vi "Insert Path Node.vi"(7 "MulticolumnListbox in":refnum<vi>, 8 "ID":i16, 9 "Node To Index Lookup Map in":map{i16, i16[]}(c390), 10 "Tree":T2[](array[typedef]), 11 "CellPosition":T1) -> (1 "Index of Selected Node":i32, 2 "Tree Out":T2[](array[typedef]), 3 "Node To Index Lookup Map out":map{i16, i16[]}(c390))   [LabVIEW 2025]
uses:
  Types/Sequencing Tree Node.ctl
  Types/Single Cmd Info.ctl
  <vilib>/picture/picture.llb/imagedata.ctl
  <vilib>/Utility/miscctls.llb/LVRowAndColumnTypeDef.ctl
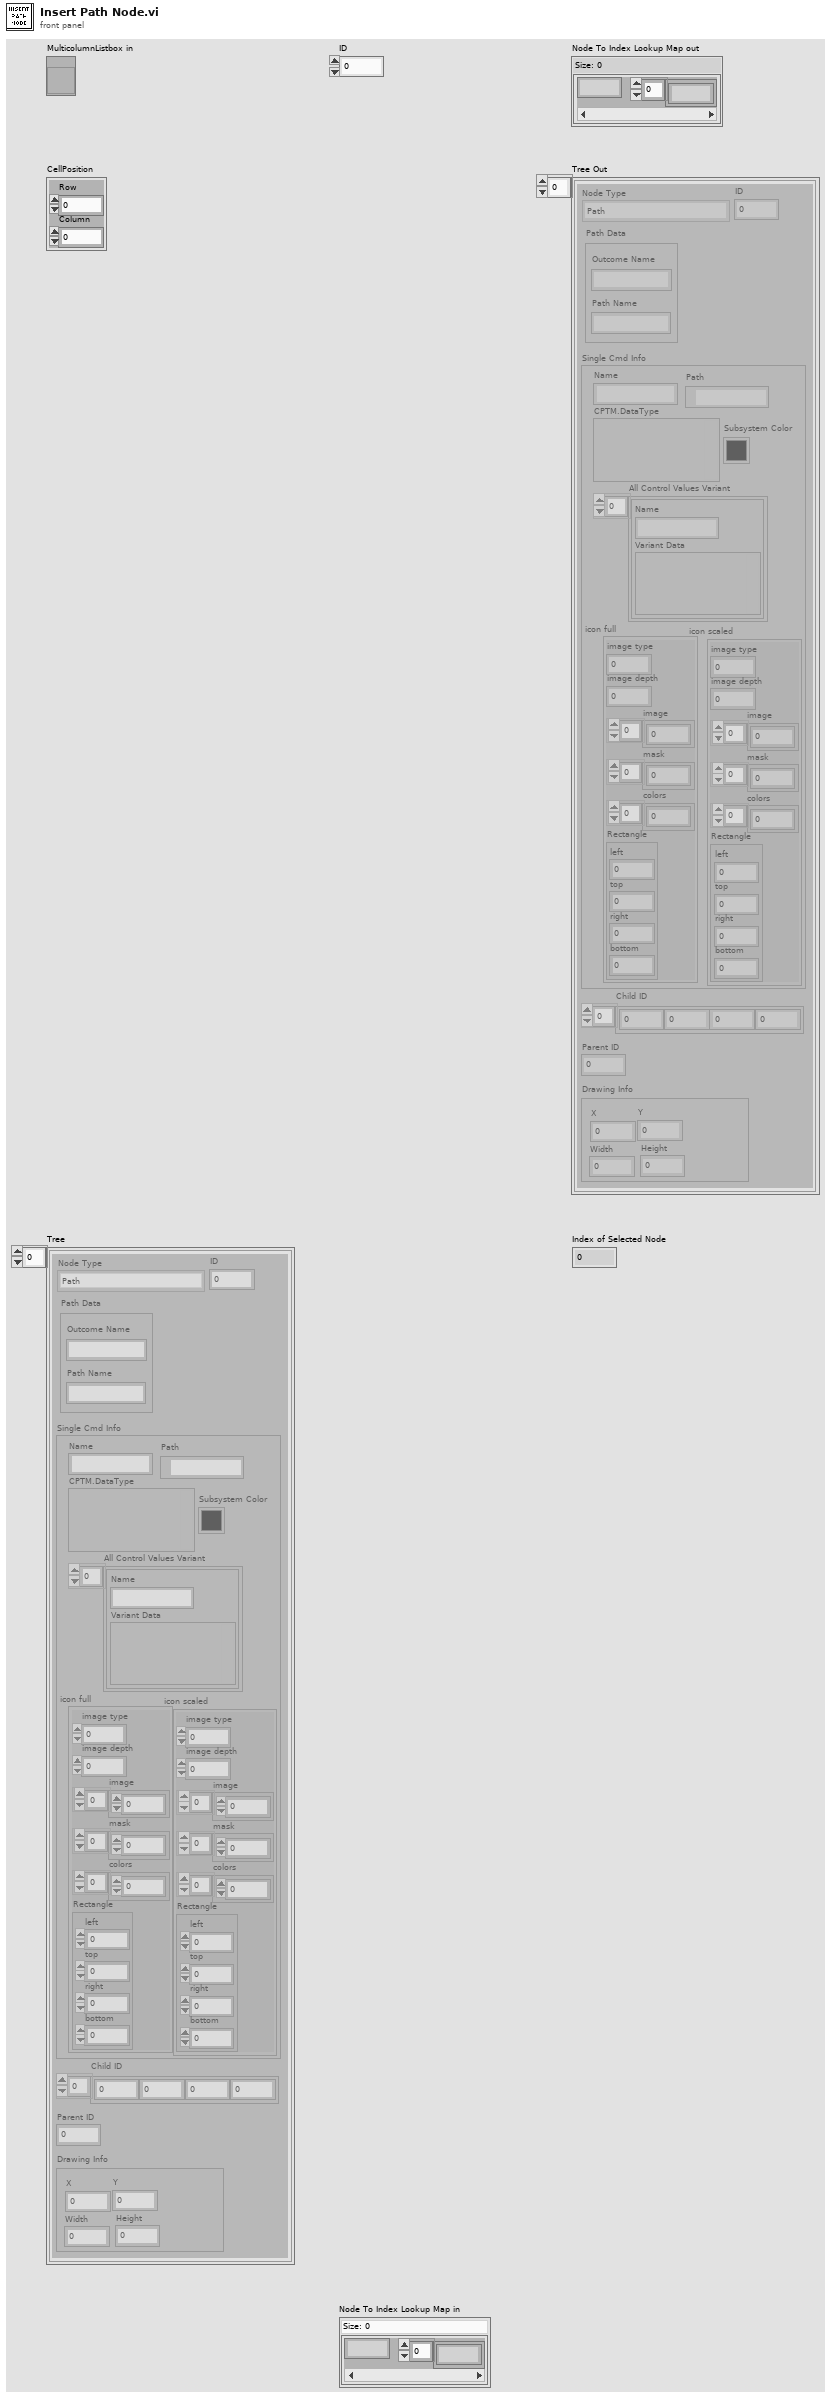
[diagram p1: front panel]
types:
  T1 = typedef "LVRowAndColumnTypeDef.ctl" = cluster{"Row":i32, "Column":i32}
  T2 = typedef "Sequencing Tree Node.ctl" = cluster{"Node Type":enum16{"Path", "Command", "Leaf"}, "ID":i16, "Path Data":cluster{"Path Name":string, "Outcome Name":string}, "Single Cmd Info":T3, "Child ID":i32[], "Parent ID":i32, "Drawing Info":cluster{"X":i32, "Y":i32, "Width":i32, "Height":i32}}
  T3 = typedef "Single Cmd Info.ctl" = cluster{"Name":string, "CPTM.DataType":variant, "All Control Values Variant":cluster{"Name":string, "Variant Data":variant}[], "icon full":T4, "icon scaled":T4, "Path":path, "Subsystem Color":u32}
  T4 = typedef "imagedata.ctl" = cluster{"image type":i32, "image depth":i32, "image":u8[], "mask":u8[], "colors":u32[], "Rectangle":cluster{"left":i16, "top":i16, "right":i16, "bottom":i16}}
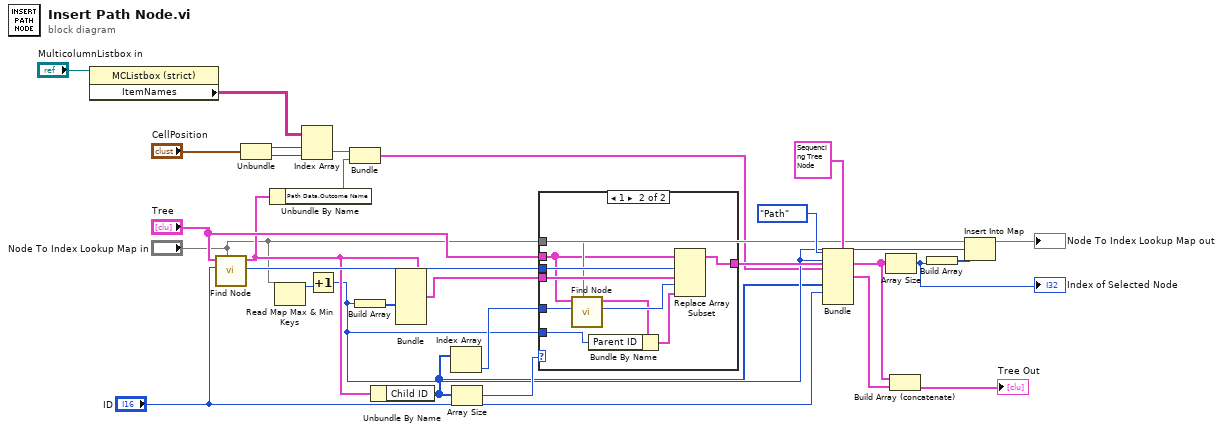
[diagram p0: block diagram]
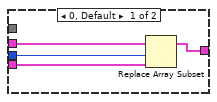
[diagram p2: hidden frame]
diagram:
  n1 = property on="Property Node" class="MCListbox (strict)"(reference="MulticolumnListbox in") -> ("ItemNames"=w12:string[][])  [unwired: 1 in, 2 out]
  n2 = call "Find Node.vi"("Node To Index Lookup Map"="Node To Index Lookup Map in", "ID"="ID", "Tree"="Tree") -> ("Index"=w10:i16, "Node"=w7:T2)  [unwired: 7 in]
  n3 = Unbundle("CellPosition") -> ("Row"=w13:i32, "Column"=w14:i32)
  n4 = Unbundle By Name(w7) -> ("Path Data.Outcome Name"=w16:string)
  n5 = Read Map Max & Min Keys(11:"Node To Index Lookup Map in") -> (3:w17:i16)  [unwired: 1 out]
  n6 = Index Array(array=w12, index (row)=w13, index (col)=w14) -> (element=w15:string)
  n7 = Increment(x=w17) -> (x+1=w3:i16)
  n8 = Bundle(w15, "Outcome Name"=w16) -> (w2:cluster{string, "Outcome Name":string})  [unwired: 1 in]
  n9 = Build Array(w3) -> (w18:i16[])
  n10 = Unbundle By Name(w7) -> ("Child ID"=w1:i32[])
  n11 = Bundle(cluster=w7, "Child ID"=w18) -> (w11:T2)  [unwired: 6 in]
  n12 = Index Array(array=w1) -> (element=w4:i32)  [unwired: 1 in]
  n13 = Array Size(array=w1) -> (size(s)=w5:i32)
  n14 = case shown="1" w5 {
    tunnel: "Tree" -> [w32 w38]
    tunnel: [w31 w42] -> w22
    tunnel: w11 -> [w30 w41]
    tunnel: w10 -> [w29 w40]
    tunnel: "Node To Index Lookup Map in" -> [_ w39]
    tunnel: w4 -> [_ w37]
    tunnel: w3 -> [_ w33]
    frame 0, Default {
      n15 = Replace Array Subset(array=w32, new element=w30, index=w29) -> (w31:T2[])
    }
    frame 1 {
      n16 = call "Find Node.vi"("Node To Index Lookup Map"=w39, "ID"=w37, "Tree"=w38) -> ("Index"=w36:i16, "Node"=w35:T2)  [unwired: 7 in]
      n17 = Bundle By Name(cluster=w35, "Parent ID"=w33) -> (w34:T2)
      n18 = Replace Array Subset(array=w38, new element #1=w41, index #1=w40, new element #2=w34, index #2=w36) -> (w42:T2[])
    }
  }
  n19 = Bundle(cluster=T2 {"Node Type"=enum."Path", "ID"=0, "Path Data"={"Path Name"="", "Outcome Name"=""}, "Single Cmd Info"={"Name"="", "CPTM.DataType"=variant, "All Control Values Variant"=[], "icon full"={"image type"=0, "image depth"=0, "image"=[], "mask"=[], "colors"=[], "Rectangle"={"left"=0, "top"=0, "right"=0, "bottom"=0}}, "icon scaled"={"image type"=0, "image depth"=0, "image"=[], "mask"=[], "colors"=[], "Rectangle"={"left"=0, "top"=0, "right"=0, "bottom"=0}}, "Path"=path "", "Subsystem Color"=0}, "Child ID"=[], "Parent ID"=0, "Drawing Info"={"X"=0, "Y"=0, "Width"=0, "Height"=0}} ("Cluster"), "Node Type"=enum16{"Path", "Command", "Leaf"}."Path", "ID"=w3, "Path Data"=w2, "Child ID"=w1, "Parent ID"="ID") -> (w23:T2)  [unwired: 2 in]
  n20 = Array Size(array=w22) -> (size(s)=w27:i32)
  "Index of Selected Node" <- w27
  n21 = Build Array (concatenate)(w22, w23) -> (→"Tree Out":T2[])
  n22 = Build Array(w27) -> (w21:i32[])
  n23 = Insert Into Map(map in="Node To Index Lookup Map in", key=w3, value=w21) -> (map out=→"Node To Index Lookup Map out":map{i16, i16[]})  [unwired: 2 out]
